vi "CH_N.vi"(6 "error in (no error)":errorcluster, 9 "Scope_pointer":u32) -> (0 "error out":errorcluster, 1 "Channel info":T1, 3 "Scope out":u32)   [LabVIEW 2018]
uses:
  LabViewHS4/libtiepie.dll
  LibTiePie.lvlib
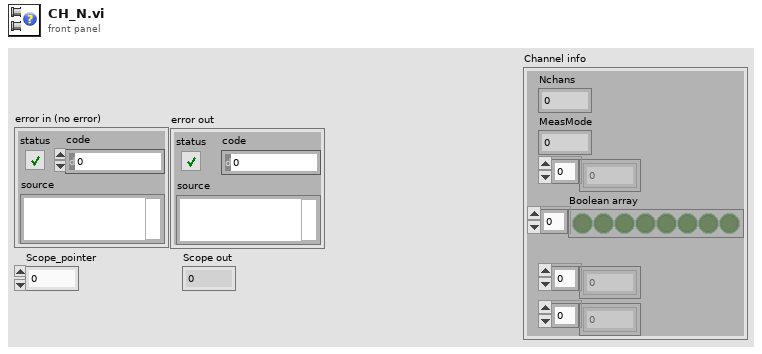
[diagram p1: front panel]
types:
  T1 = cluster{"Nchans":u16, "MeasMode":u32, dbl[], "Boolean array":bool[], u32[], dbl[]}
  T2 = cluster{"Nchans":u16, "MeasMode":u32, dbl[], bool[], u32[], dbl[]}
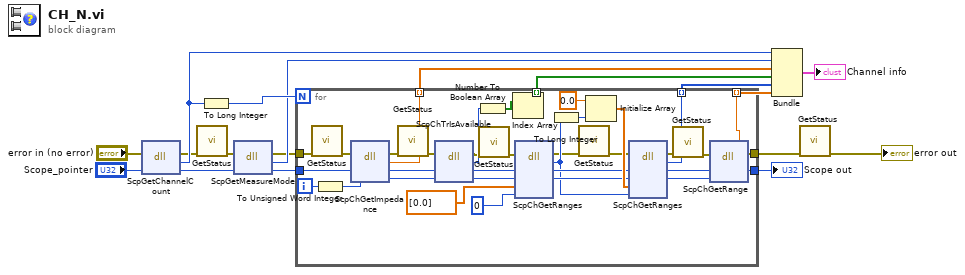
[diagram p0: block diagram]
diagram:
  n1 = dll-call lib="C:/Users/cwaha/Documents/LabViewHS4/libtiepie.dll" fn="ScpGetChannelCount"(error in="error in (no error)", "Scope_pointer"="Scope_pointer") -> (error out=w6:errorcluster, "Nchans"=w13:u16, "Scope_pointer"=w15:u32)  [unwired: 2 in, 1 out]
  n2 = call "GetStatus.vi"("error in (no error)"=w6) -> ("error out"=w7:errorcluster)  [unwired: 10 in]
  n3 = To Long Integer(number=w13) -> (32bit integer=w16:i32)
  n4 = dll-call lib="C:/Users/cwaha/Documents/LabViewHS4/libtiepie.dll" fn="ScpGetMeasureMode"(error in=w7, "OSC?id"=w15) -> (error out=w5:errorcluster, "MeasMode"=w12:u32, "OSC?id"=w14:u32)  [unwired: 2 in, 1 out]
  n5 = for {
    N: w16 -> [_]
    tunnel: w14 -> [w53]
    tunnel: w5 -> [w30]
    tunnel: [w34] -> w4
    tunnel: [w32] -> w11
    tunnel: [w38] -> w10 mode=indexing
    tunnel: [w33] -> w9 mode=indexing
    tunnel: [w35] -> w8 mode=indexing
    tunnel: [w19] -> w1 mode=indexing
    i -> [w50]
    n6 = call "GetStatus.vi"("error in (no error)"=w30) -> ("error out"=w29:errorcluster)  [unwired: 10 in]
    n7 = To Unsigned Word Integer(number=w50) -> (unsigned 16bit integer=w49:u16)
    n8 = dll-call lib="C:/Users/cwaha/Documents/LabViewHS4/libtiepie.dll" fn="ScpChGetImpedance"(error in=w29, "osc"=w53, "ch"=w49) -> (error out=w28:errorcluster, "IMP"=w38:dbl, "osc"=w52:u32, "ch"=w51:u16)  [unwired: 2 in, 1 out]
    n9 = call "GetStatus.vi"("error in (no error)"=w28) -> ("error out"=w27:errorcluster)  [unwired: 10 in]
    n10 = dll-call lib="C:/Users/cwaha/Documents/LabViewHS4/libtiepie.dll" fn="ScpChTrIsAvailable"(error in=w27, "OSC_id"=w52, "CH_id"=w51) -> (error out=w26:errorcluster, "TRIG?"=w31:u8, "OSC_id"=w48:u32, "CH_id"=w47:u16)  [unwired: 2 in, 1 out]
    n11 = Number To Boolean Array(number=w31) -> (Boolean array=w20:bool[])
    n12 = call "GetStatus.vi"("error in (no error)"=w26) -> ("error out"=w25:errorcluster)  [unwired: 10 in]
    n13 = Index Array(array=w20) -> (element=w19:bool)  [unwired: 1 in]
    n14 = dll-call lib="C:/Users/cwaha/Documents/LabViewHS4/libtiepie.dll" fn="ScpChGetRanges"(error in=w25, "OSC_ID"=w48, "CH"=w47, "NULL"=dbl[] [0.0], "rng"=u32 0 ("NULL")) -> (error out=w24:errorcluster, "RNG"=w41:u32, "OSC_ID"=w42:u32, "CH"=w43:u16)  [unwired: 4 in, 1 out]
    n15 = To Long Integer(number=w41) -> (32bit integer=w46:i32)
    n16 = call "GetStatus.vi"("error in (no error)"=w24) -> ("error out"=w23:errorcluster)  [unwired: 10 in]
    n17 = Initialize Array(0.0 ("element"), w46) -> (w44:dbl[])
    n18 = dll-call lib="C:/Users/cwaha/Documents/LabViewHS4/libtiepie.dll" fn="ScpChGetRanges"(error in=w23, "OSC_ID"=w42, "CH"=w43, "NULL"=w44, "rng"=w41) -> (error out=w22:errorcluster, "RNGS"=w33:u32, "OSC_ID"=w37:u32, "CH"=w36:u16)  [unwired: 4 in, 1 out]
    n19 = call "GetStatus.vi"("error in (no error)"=w22) -> ("error out"=w21:errorcluster)  [unwired: 10 in]
    n20 = dll-call lib="C:/Users/cwaha/Documents/LabViewHS4/libtiepie.dll" fn="ScpChGetRange"(error in=w21, "Osc_ID"=w37, "CH_ID"=w36) -> (error out=w34:errorcluster, "RNG"=w35:dbl, "Osc_ID"=w32:u32)  [unwired: 3 in, 1 out]
  }
  "Scope out" <- w11
  n21 = Bundle("Nchans"=w13, "MeasMode"=w12, w10, w1, w9, w8) -> (→"Channel info":T2)  [unwired: 1 in]
  n22 = call "GetStatus.vi"("error in (no error)"=w4) -> ("error out"=→"error out":errorcluster)  [unwired: 10 in]
